vi "Try Match Response.vi"(8 "error in":errorcluster, 10 "ICAN CC Frame":refnum<class "ICAN CC Frame.lvclass">, 11 "SDO Transfer in":refnum<class "SDO Transfer.lvclass">) -> (0 "error out":errorcluster, 2 "Success":bool, 3 "SDO Transfer out":refnum<class "SDO Transfer.lvclass">)   [LabVIEW 2020, in "SDO Manager.lvlib" / "SDO Transfer.lvclass"]
uses:
  SDO Transfer.lvclass
  HAL/Source/Interfaces/ICAN CC Frame/ICAN CC Frame.lvclass
  SDO Transfer.lvclass/SDO Transfer.ctl
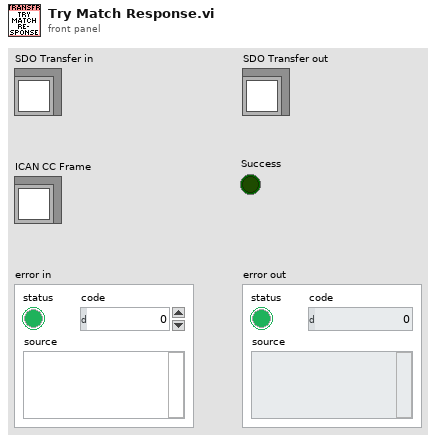
[diagram p1: front panel]
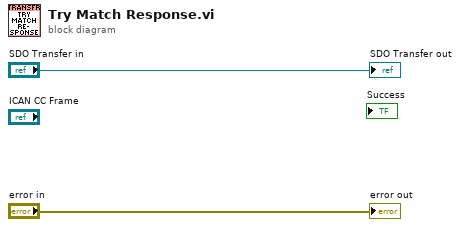
[diagram p0: block diagram]
diagram:
  "SDO Transfer out" <- "SDO Transfer in"
  "error out" <- "error in"
